vi "stop_on_notification.vi"(1 "notifier out":refnum<notifier>) -> (0 "Boolean":bool)   [LabVIEW 2010]
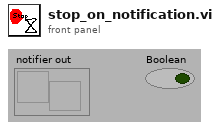
[diagram p1: front panel]
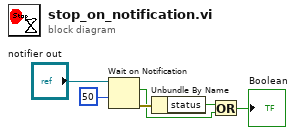
[diagram p0: block diagram]
diagram:
  n1 = Wait on Notification(notifier="notifier out", timeout in ms (-1)=50) -> (notification=w1:bool, error out=w2:errorcluster)  [unwired: 2 in, 2 out]
  n2 = Unbundle By Name(w2) -> ("status"=w4:bool)
  n3 = Or(x=w4, y=w1) -> (x .or. y?=→"Boolean":bool)
